vi "多线程发送配置.vi"() -> ()   [LabVIEW 2016]
uses:
  <vilib>/Utility/miscctls.llb/LVPointTypeDef.ctl
  <vilib>/Averna/Notify Icon/NotifyIcon.llb/BalloonIcon.ctl
  <vilib>/Utility/config.llb/Write Key (Boolean).vi
  <vilib>/Utility/config.llb/Read Key (Boolean).vi
  <vilib>/Averna/Notify Icon/NotifyIcon.llb/GetSelectedItemEvent.vi
  <vilib>/Averna/Notify Icon/NotifyIcon.llb/SetVisible.vi
  <vilib>/Averna/Notify Icon/NotifyIcon.llb/SetMenuDefaultItem.vi
  <vilib>/Averna/Notify Icon/NotifyIcon.llb/SetTipText.vi
  <vilib>/Utility/config.llb/NI_LVConfig.lvlib
  <vilib>/Averna/Notify Icon/NotifyIcon.llb/NotifyIcon.lvclass
panel:
  out "error out":errorcluster
  in  "停止 2":bool
  in  "线程选用配置":cluster{"线程1":bool, "线程2":bool, "线程3":bool}
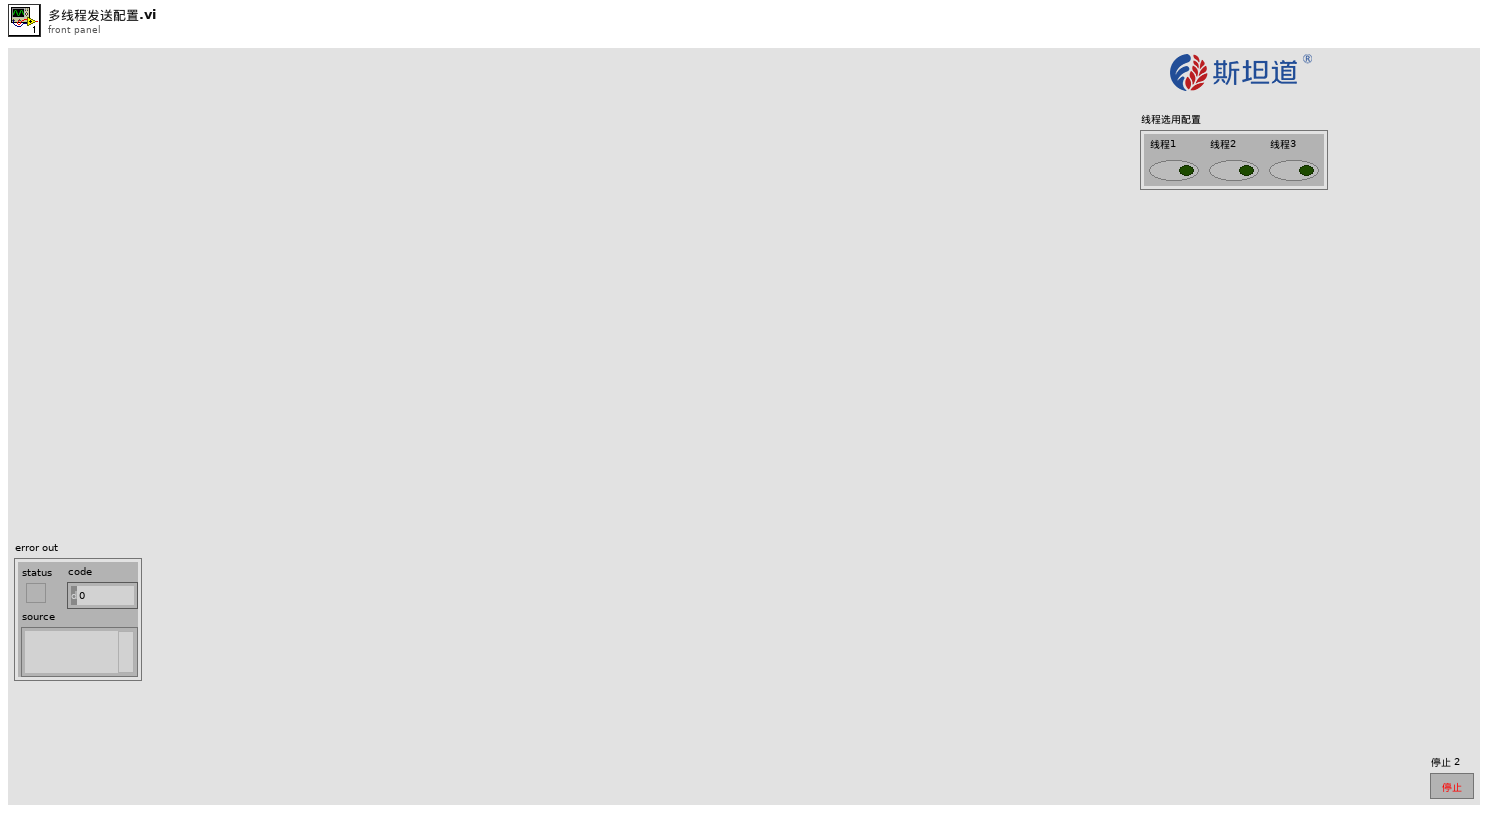
[diagram p1: front panel]
types:
  T1 = typedef "LVPointTypeDef.ctl" = cluster{"Horizontal":i16, "Vertical":i16}
  T2 = enum32{"invalid app kind", "Development System", "Run Time System", "Student Edition", "Embedded LabVIEW", "Evaluation", "Custom"}
  T3 = enum32{"Invalid", "Standard", "Closed", "Hidden", "Minimized", "Maximized"}
  T4 = typedef "NI_LVConfig.lvlib/Config Data RefNum.ctl" = refnum<k1>
  T5 = typedef "NotifyIcon.lvlib/NotifyIcon.lvclass/BalloonIcon.ctl" = enum32{"None", "Information", "Warning", "Error"}
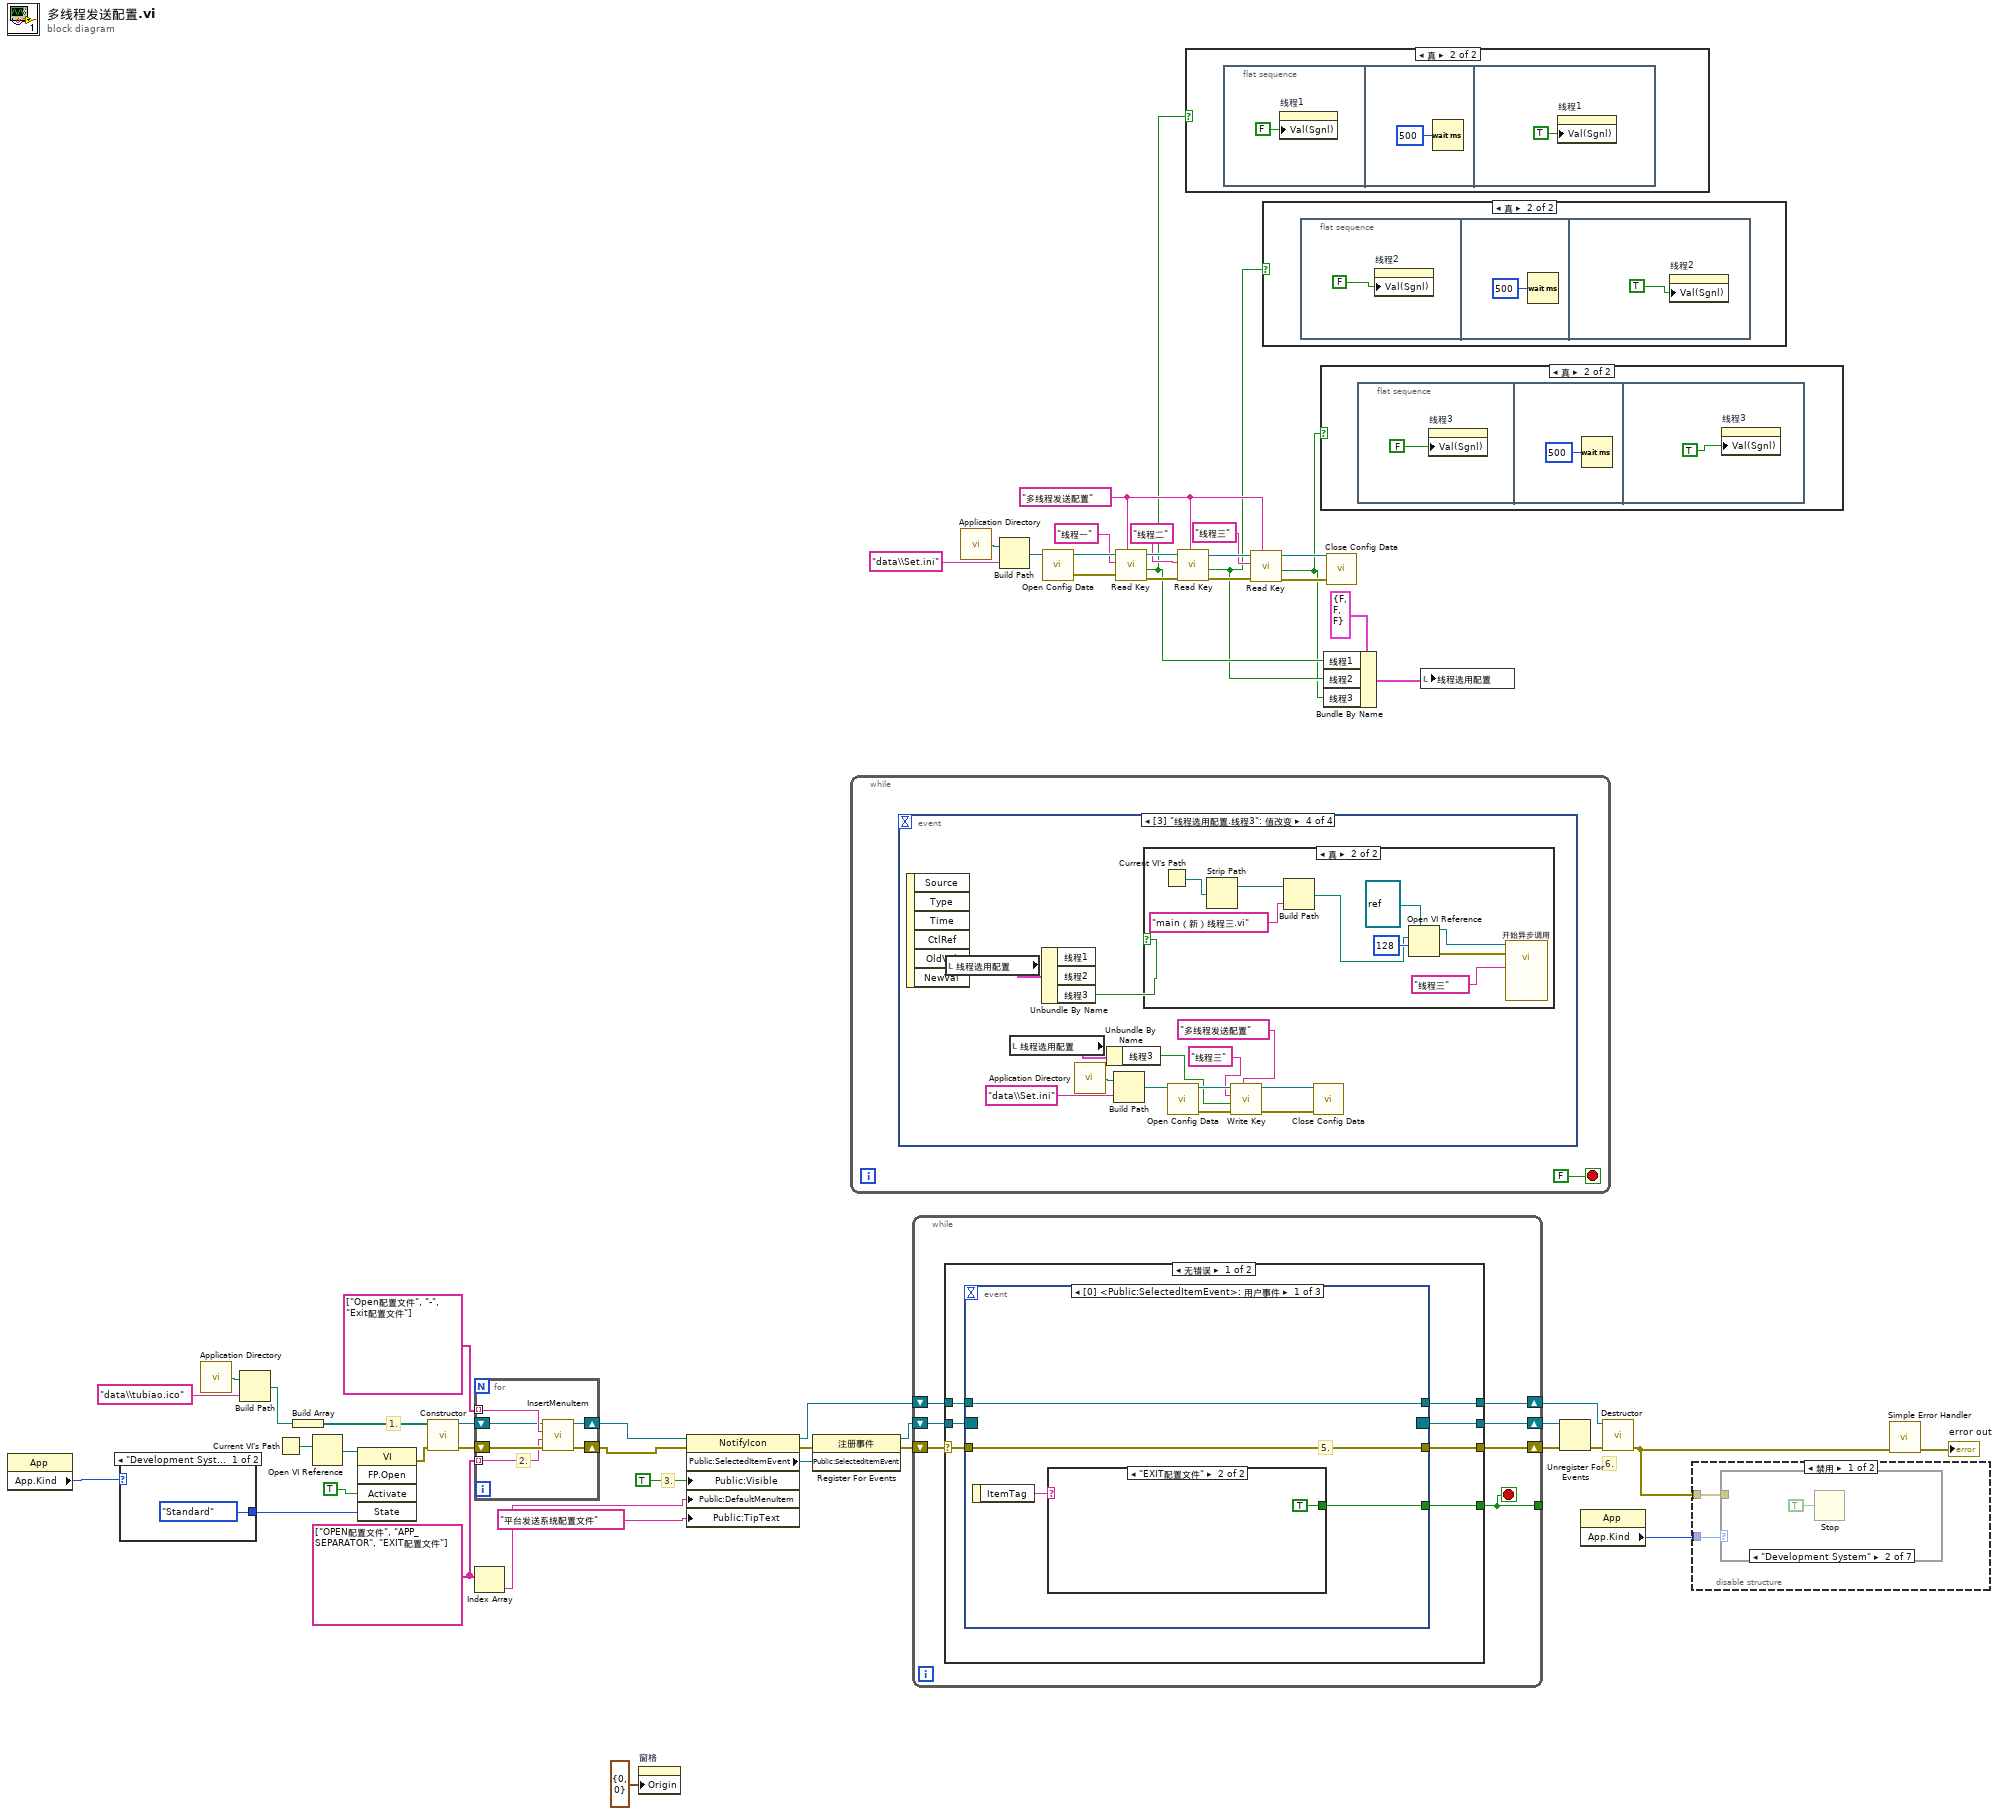
[diagram p0: block diagram]
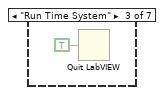
[diagram p3: hidden frame]
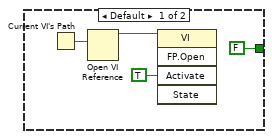
[diagram p9: hidden frame]
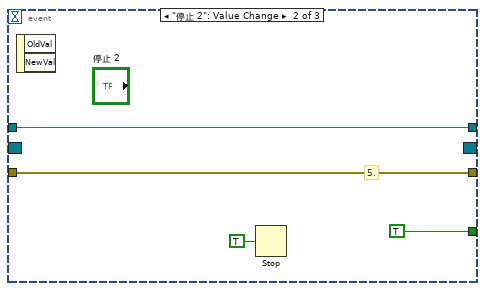
[diagram p10: hidden frame]
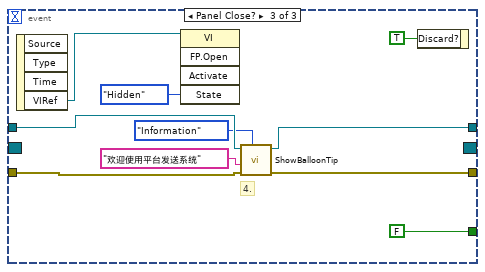
[diagram p11: hidden frame]
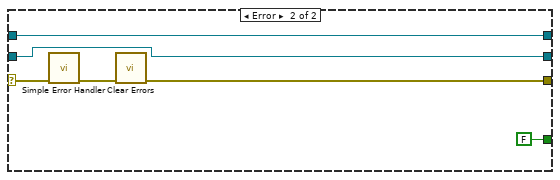
[diagram p12: hidden frame]
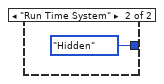
[diagram p13: hidden frame]
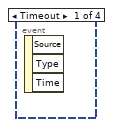
[diagram p17: hidden frame]
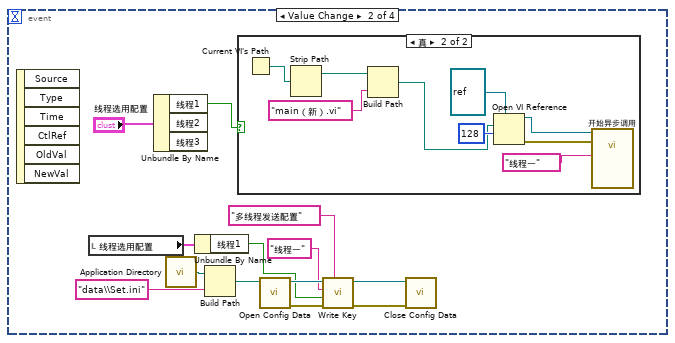
[diagram p18: hidden frame]
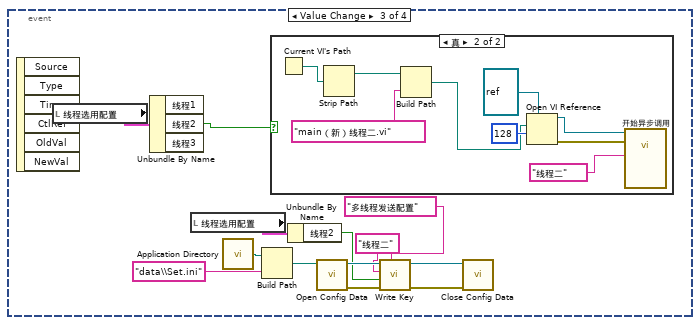
[diagram p20: hidden frame]
diagram:
  w24 = string[] ["OPEN配置文件", "APP_SEPARATOR", "EXIT配置文件"]
  w41 = "多线程发送配置" ("section")
  # "6."
  # "3."
  # "1."
  n1 = property class="App"() -> ("App.Kind"=w32:T2)  [unwired: 2 in, 2 out]
  n2 = case shown="\"Development System\", 默认" w32 {
    tunnel: [T3."Standard" ("状态") T3."Hidden" ("状态")] -> w4
    frame "Development System", Default {
    }
    frame "Run Time System" {
    }
  }
  n3 = call <vilib>:"Application Directory.vi"() -> ("Application Directory"=w26:path)
  n4 = Build Path(base path=w26, name or relative path="data\\tubiao.ico" ("名称或相对路径")) -> (appended path=w16:path)
  n5 = Current VI's Path() -> (path=w29:path)
  n6 = Build Array(w16) -> (w21:path[])
  n7 = Open VI Reference(vi path=w29) -> (vi reference=w30:refnum<vi>)  [unwired: 5 in, 1 out]
  n8 = invoke class="VI" method="FP.Open"(reference=w30, "Activate"=TRUE ("激活？"), "State"=w4) -> (error out=w31:errorcluster)  [unwired: 2 in, 4 out]
  n9 = call <vilib>:"Constructor.vi"("error in"=w31, "IconFilePathList"=w21) -> ("error out"=w17:errorcluster, "NotifyIcon"=w25:refnum<class "NotifyIcon.lvclass">)  [unwired: 8 in]
  n10 = for {
    shift-right: [w59] -> w2
    shift-left: w17 -> [w60]
    tunnel: string[] ["Open配置文件", "-", "Exit配置文件"] -> [w58] mode=indexing
    tunnel: w24 -> [w57] mode=indexing
    shift-right: [w55] -> w3
    shift-left: w25 -> [w56]
    # "2."
    n11 = call <vilib>:"InsertMenuItem.vi"("error in"=w60, "ItemTag"=w57, "ItemName"=w58, "NotifyIcon in"=w56) -> ("error out"=w59:errorcluster, "NotifyIcon out"=w55:refnum<class "NotifyIcon.lvclass">)  [unwired: 6 in]
  }
  n12 = Index Array(array=w24) -> (element=w23:string)  [unwired: 1 in]
  n13 = property on="窗格" class="Pane"("Origin"=T1 {"Horizontal"=0, "Vertical"=0} ("原点")) -> ()  [unwired: 2 in, 2 out]
  n14 = property class="NotifyIcon"(reference=w3, error in=w2, "Public:Visible"=TRUE ("Visible"), "Public:DefaultMenuItem"=w23, "Public:TipText"="平台发送系统配置文件" ("TipText")) -> (reference out=w8:refnum<class "NotifyIcon.lvclass">, error out=w18:errorcluster, "Public:SelectedItemEvent"=w19:refnum<user-event>)
  n15 = register-events(error in=w18, w19) -> (reference out=w7:refnum<event-registration>, error out=w6:errorcluster)  [unwired: 1 in]
  n16 = while {
    stop <- FALSE stop-if-true
    n17 = event shown="[3] \"线程选用配置.线程3\": 值改变" {
      selector: _ -> [_ _ _ _]
      dyn-events: _ -> [_ _ _ _]
      timeout: _ -> [_ _ _ _]
      event Timeout {
        n18 = event-data() -> ()  [unwired: 1 in, 3 out]
      }
      event "线程选用配置.线程1": Value Change {
        n19 = event-data() -> ()  [unwired: 1 in, 6 out]
        n20 = local read "线程选用配置"() -> (w63:cluster{"线程1":bool, "线程2":bool, "线程3":bool})
        n21 = Unbundle By Name("线程选用配置") -> ("线程1"=w73:bool)  [unwired: 2 out]
        n22 = call <vilib>:"Application Directory.vi"() -> ("Application Directory"=w66:path)
        n23 = Unbundle By Name(w63) -> ("线程1"=w62:bool)
        n24 = Build Path(base path=w66, name or relative path="data\\Set.ini" ("名称或相对路径")) -> (appended path=w68:path)
        n25 = case shown="真" w73 {
          frame False {
          }
          frame True {
            n26 = Current VI's Path() -> (path=w78:path)
            n27 = Strip Path(path=w78) -> (stripped path=w77:path)  [unwired: 1 out]
            n28 = Build Path(base path=w77, name or relative path="main（新）.vi" ("名称或相对路径")) -> (appended path=w75:path)
            n29 = Open VI Reference(type specifier VI Refnum (for type only)=refnum<vi> refnum ("类型说明符VI引用句柄（仅用于类型）"), vi path=w75, options=128 ("选项")) -> (vi reference=w82:refnum<vi>, error out=w81:errorcluster)  [unwired: 3 in]
            n30 = call-by-ref "开始异步调用"(reference=w82, error in=w81, "线程选择"="线程一") -> ()  [unwired: 11 in, 2 out]
          }
        }
        n31 = call <vilib>:"Open Config Data.vi"("configuration file path"=w68) -> ("error out"=w70:errorcluster, "refnum"=w69:T4)  [unwired: 8 in, 1 out]
        n32 = call-poly <vilib>:"Write Key.vi"("section"="多线程发送配置", "error in (no error)"=w70, "value"=w62, "key"="线程一", "refnum"=w69) -> ("error out"=w72:errorcluster, "refnum out"=w71:T4)  [unwired: 4 in, 1 out]
        n33 = call <vilib>:"Close Config Data.vi"("error in (no error)"=w72, "refnum"=w71) -> ()  [unwired: 8 in, 2 out]
      }
      event "线程选用配置.线程2": Value Change {
        n34 = event-data() -> ()  [unwired: 1 in, 6 out]
        n35 = local read "线程选用配置"() -> (w95:cluster{"线程1":bool, "线程2":bool, "线程3":bool})
        n36 = Unbundle By Name(w95) -> ("线程2"=w96:bool)  [unwired: 2 out]
        n37 = local read "线程选用配置"() -> (w87:cluster{"线程1":bool, "线程2":bool, "线程3":bool})
        n38 = call <vilib>:"Application Directory.vi"() -> ("Application Directory"=w88:path)
        n39 = Build Path(base path=w88, name or relative path="data\\Set.ini" ("名称或相对路径")) -> (appended path=w90:path)
        n40 = case shown="真" w96 {
          frame False {
          }
          frame True {
            n41 = Current VI's Path() -> (path=w100:path)
            n42 = Strip Path(path=w100) -> (stripped path=w99:path)  [unwired: 1 out]
            n43 = Build Path(base path=w99, name or relative path="main（新）线程二.vi" ("名称或相对路径")) -> (appended path=w97:path)
            n44 = Open VI Reference(type specifier VI Refnum (for type only)=refnum<vi> refnum ("类型说明符VI引用句柄（仅用于类型）"), vi path=w97, options=128 ("选项")) -> (vi reference=w104:refnum<vi>, error out=w103:errorcluster)  [unwired: 3 in]
            n45 = call-by-ref "开始异步调用"(reference=w104, error in=w103, "线程选择"="线程二") -> ()  [unwired: 11 in, 2 out]
          }
        }
        n46 = Unbundle By Name(w87) -> ("线程2"=w86:bool)
        n47 = call <vilib>:"Open Config Data.vi"("configuration file path"=w90) -> ("error out"=w92:errorcluster, "refnum"=w91:T4)  [unwired: 8 in, 1 out]
        n48 = call-poly <vilib>:"Write Key.vi"("section"="多线程发送配置", "error in (no error)"=w92, "value"=w86, "key"="线程二", "refnum"=w91) -> ("error out"=w94:errorcluster, "refnum out"=w93:T4)  [unwired: 4 in, 1 out]
        n49 = call <vilib>:"Close Config Data.vi"("error in (no error)"=w94, "refnum"=w93) -> ()  [unwired: 8 in, 2 out]
      }
      event "线程选用配置.线程3": Value Change {
        n50 = event-data() -> ()  [unwired: 1 in, 6 out]
        n51 = local read "线程选用配置"() -> (w118:cluster{"线程1":bool, "线程2":bool, "线程3":bool})
        n52 = local read "线程选用配置"() -> (w109:cluster{"线程1":bool, "线程2":bool, "线程3":bool})
        n53 = Unbundle By Name(w118) -> ("线程3"=w117:bool)  [unwired: 2 out]
        n54 = call <vilib>:"Application Directory.vi"() -> ("Application Directory"=w110:path)
        n55 = Unbundle By Name(w109) -> ("线程3"=w106:bool)
        n56 = Build Path(base path=w110, name or relative path="data\\Set.ini" ("名称或相对路径")) -> (appended path=w112:path)
        n57 = case shown="真" w117 {
          frame False {
          }
          frame True {
            n58 = Current VI's Path() -> (path=w122:path)
            n59 = Strip Path(path=w122) -> (stripped path=w121:path)  [unwired: 1 out]
            n60 = Build Path(base path=w121, name or relative path="main（新）线程三.vi" ("名称或相对路径")) -> (appended path=w119:path)
            n61 = Open VI Reference(type specifier VI Refnum (for type only)=refnum<vi> refnum ("类型说明符VI引用句柄（仅用于类型）"), vi path=w119, options=128 ("选项")) -> (vi reference=w126:refnum<vi>, error out=w125:errorcluster)  [unwired: 3 in]
            n62 = call-by-ref "开始异步调用"(reference=w126, error in=w125, "线程选择"="线程三") -> ()  [unwired: 11 in, 2 out]
          }
        }
        n63 = call <vilib>:"Open Config Data.vi"("configuration file path"=w112) -> ("error out"=w114:errorcluster, "refnum"=w113:T4)  [unwired: 8 in, 1 out]
        n64 = call-poly <vilib>:"Write Key.vi"("section"="多线程发送配置", "error in (no error)"=w114, "value"=w106, "key"="线程三", "refnum"=w113) -> ("error out"=w116:errorcluster, "refnum out"=w115:T4)  [unwired: 4 in, 1 out]
        n65 = call <vilib>:"Close Config Data.vi"("error in (no error)"=w116, "refnum"=w115) -> ()  [unwired: 8 in, 2 out]
      }
    }
  }
  n66 = while {
    shift-right: [w131] -> w10
    shift-left: w6 -> [w130]
    shift-right: [w132] -> w13
    shift-left: w8 -> [w133]
    shift-right: [w129] -> w12
    shift-left: w7 -> [w134]
    tunnel: [w128] -> _
    stop <- w128 stop-if-true
    n67 = case shown="无错误" w130 {
      selector: w130 -> [w136 w170]
      tunnel: w134 -> [w141 w165]
      tunnel: w133 -> [w140 w166]
      tunnel: [w139 w166] -> w132
      tunnel: [w138 w168] -> w131
      tunnel: [w137 FALSE ("Discard?")] -> w128
      tunnel: [w135 w165] -> w129
      frame No Error {
        n68 = event shown="[0] <Public:SelectedItemEvent>: 用户事件" {
          selector: w141 -> [_ _ _]
          dyn-events: [_ _ _] -> w135
          timeout: _ -> [_ _ _]
          tunnel: w136 -> [w144 w154 w163]
          tunnel: [w144 w154 w162] -> w138
          tunnel: [w143 TRUE FALSE ("Discard?")] -> w137
          tunnel: w140 -> [w142 w152 w164]
          tunnel: [w142 w152 w161] -> w139
          event User Event {
            # "5."
            n69 = event-data() -> ("ItemTag"=w145:string)  [unwired: 1 in]
            n70 = case shown="\"EXIT配置文件\"" w145 {
              tunnel: [FALSE TRUE] -> w143
              frame Default {
                n71 = Current VI's Path() -> (path=w146:path)
                n72 = Open VI Reference(vi path=w146) -> (vi reference=w147:refnum<vi>)  [unwired: 5 in, 1 out]
                n73 = invoke class="VI" method="FP.Open"(reference=w147, "Activate"=TRUE ("激活？")) -> ()  [unwired: 3 in, 5 out]
              }
              frame "EXIT配置文件" {
              }
            }
          }
          event "停止 2": Value Change {
            # "5."
            n74 = event-data() -> ()  [unwired: 1 in, 2 out]
            n75 = Stop(stop? (T)=TRUE ("可见")) -> ()
          }
          event Panel Close? {
            # "4."
            n76 = event-data() -> ("VIRef"=w157:refnum<vi>)  [unwired: 1 in, 3 out]
            n77 = invoke class="VI" method="FP.Open"(reference=w157, "State"=T3."Hidden" ("状态")) -> ()  [unwired: 3 in, 5 out]
            n78 = call <vilib>:"ShowBalloonTip.vi"("Balloon Icon"=BalloonIcon."Information", "error in"=w163, "Text"="欢迎使用平台发送系统", "NotifyIcon in"=w164) -> ("error out"=w162:errorcluster, "NotifyIcon out"=w161:refnum<class "NotifyIcon.lvclass">)  [unwired: 6 in]
            n79 = event-data("Discard?"=TRUE ("放弃？")) -> ()  [unwired: 1 in, 1 out]
          }
        }
      }
      frame Error {
        n80 = call <vilib>:"Simple Error Handler.vi"("error in (no error)"=w170) -> ("error out"=w169:errorcluster)  [unwired: 4 in, 4 out]
        n81 = call <vilib>:"Clear Errors.vi"("error in (no error)"=w169) -> ("error out"=w168:errorcluster)  [unwired: 5 in, 1 out]
      }
    }
  }
  n82 = call <vilib>:"Application Directory.vi"() -> ("Application Directory"=w52:path)
  n83 = Build Path(base path=w52, name or relative path="data\\Set.ini" ("名称或相对路径")) -> (appended path=w50:path)
  n84 = call <vilib>:"Open Config Data.vi"("configuration file path"=w50) -> ("error out"=w48:errorcluster, "refnum"=w49:T4)  [unwired: 8 in, 1 out]
  n85 = call-poly <vilib>:"Read Key.vi"("section"=w41, "error in (no error)"=w48, "key"="线程一", "refnum"=w49) -> ("error out"=w46:errorcluster, "value"=w35:bool, "refnum out"=w47:T4)  [unwired: 4 in, 1 out]
  n86 = call-poly <vilib>:"Read Key.vi"("section"=w41, "error in (no error)"=w46, "key"="线程二", "refnum"=w47) -> ("error out"=w44:errorcluster, "value"=w34:bool, "refnum out"=w45:T4)  [unwired: 4 in, 1 out]
  n87 = case shown="真" w35 {
    frame False {
    }
    frame True {
      n88 = flat-sequence {
        frame #0 {
          n89 = property on="线程1" class="Bool (严格)"("Val(Sgnl)"=FALSE ("值(信号)")) -> ()  [unwired: 2 in, 2 out]
        }
        frame #1 {
          n90 = Wait (ms)(milliseconds to wait=u32 500 ("等待时间（毫秒）")) -> ()  [unwired: 1 out]
        }
        frame #2 {
          n91 = property on="线程1" class="Bool (严格)"("Val(Sgnl)"=TRUE ("值(信号)")) -> ()  [unwired: 2 in, 2 out]
        }
      }
    }
  }
  n92 = call-poly <vilib>:"Read Key.vi"("section"=w41, "error in (no error)"=w44, "key"="线程三", "refnum"=w45) -> ("error out"=w42:errorcluster, "value"=w33:bool, "refnum out"=w43:T4)  [unwired: 4 in, 1 out]
  n93 = case shown="真" w34 {
    frame False {
    }
    frame True {
      n94 = flat-sequence {
        frame #0 {
          n95 = property on="线程2" class="Bool (严格)"("Val(Sgnl)"=FALSE ("值(信号)")) -> ()  [unwired: 2 in, 2 out]
        }
        frame #1 {
          n96 = Wait (ms)(milliseconds to wait=u32 500 ("等待时间（毫秒）")) -> ()  [unwired: 1 out]
        }
        frame #2 {
          n97 = property on="线程2" class="Bool (严格)"("Val(Sgnl)"=TRUE ("值(信号)")) -> ()  [unwired: 2 in, 2 out]
        }
      }
    }
  }
  n98 = case shown="真" w33 {
    frame False {
    }
    frame True {
      n99 = flat-sequence {
        frame #0 {
          n100 = property on="线程3" class="Bool (严格)"("Val(Sgnl)"=FALSE ("值(信号)")) -> ()  [unwired: 2 in, 2 out]
        }
        frame #1 {
          n101 = Wait (ms)(milliseconds to wait=u32 500 ("等待时间（毫秒）")) -> ()  [unwired: 1 out]
        }
        frame #2 {
          n102 = property on="线程3" class="Bool (严格)"("Val(Sgnl)"=TRUE ("值(信号)")) -> ()  [unwired: 2 in, 2 out]
        }
      }
    }
  }
  n103 = Bundle By Name(cluster=cluster{"线程1":bool, "线程2":bool, "线程3":bool} {"线程1"=FALSE, "线程2"=FALSE, "线程3"=FALSE} ("线程选用配置"), "线程1"=w35, "线程2"=w34, "线程3"=w33) -> (w36:cluster{"线程1":bool, "线程2":bool, "线程3":bool})
  n104 = call <vilib>:"Close Config Data.vi"("error in (no error)"=w42, "refnum"=w43) -> ()  [unwired: 8 in, 2 out]
  n105 = local write "线程选用配置"(w36) -> ()
  n106 = Unregister For Events(event registration refnum=w12, error in=w10) -> (error out=w9:errorcluster)
  n107 = property class="App"() -> ("App.Kind"=w14:T2)  [unwired: 2 in, 2 out]
  n108 = call <vilib>:"Destructor.vi"("error in"=w9, "NotifyIcon"=w13) -> ("error out"=w15:errorcluster)  [unwired: 9 in]
  n109 = disable-structure shown="禁用" {
    disable-tunnel: w15 -> [w181 _]
    disable-tunnel: w14 -> [w180 _]
    frame Disabled {
      n110 = case shown="\"Development System\"" w180 {
        tunnel: w181 -> [_ _ _ _ _ _ _]
        frame "invalid app kind", Default {
        }
        frame "Development System" {
          n111 = Stop(stop? (T)=TRUE ("可见")) -> ()
        }
        frame "Run Time System" {
          n112 = Quit LabVIEW(quit? (T)=TRUE ("退出？(T)")) -> ()
        }
        frame "Student Edition" {
        }
        frame "Embedded LabVIEW" {
        }
        frame "Evaluation" {
        }
        frame "Custom" {
        }
      }
    }
    frame Enabled {
    }
  }
  n113 = call <vilib>:"Simple Error Handler.vi"("error in (no error)"=w15) -> ("error out"=→"error out":errorcluster)  [unwired: 4 in, 4 out]
